vi "git resolve conflicts command.vi"(10 "Choosen file":string, 11 "ours vi path":path) -> (2 "git stage file and resolve conflict":string, 3 "git checkout selected file cmd":string)   [LabVIEW 2022 SP3]
panel:
  # "This is the path of the repository on which we are resolving conflicts. In this path needs to be \"ours\" repository."
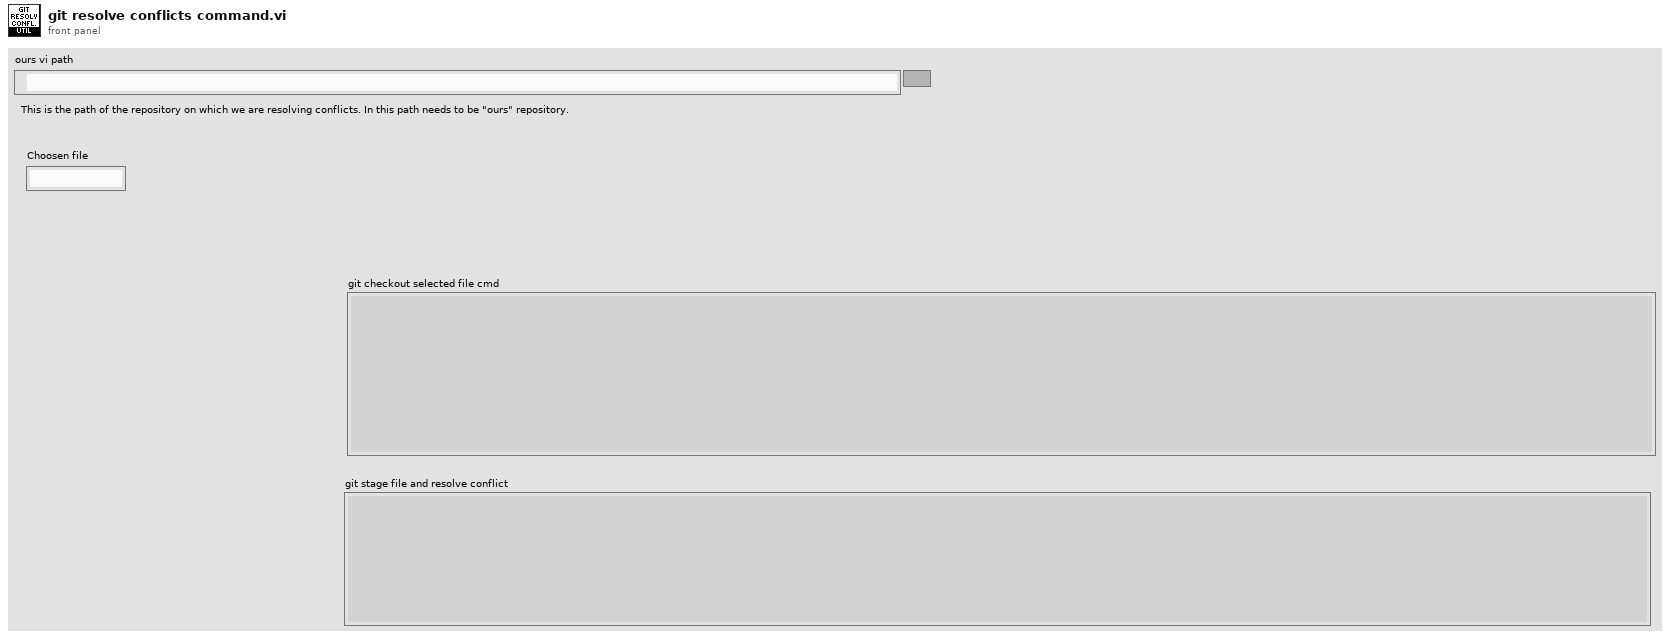
[diagram p1: front panel]
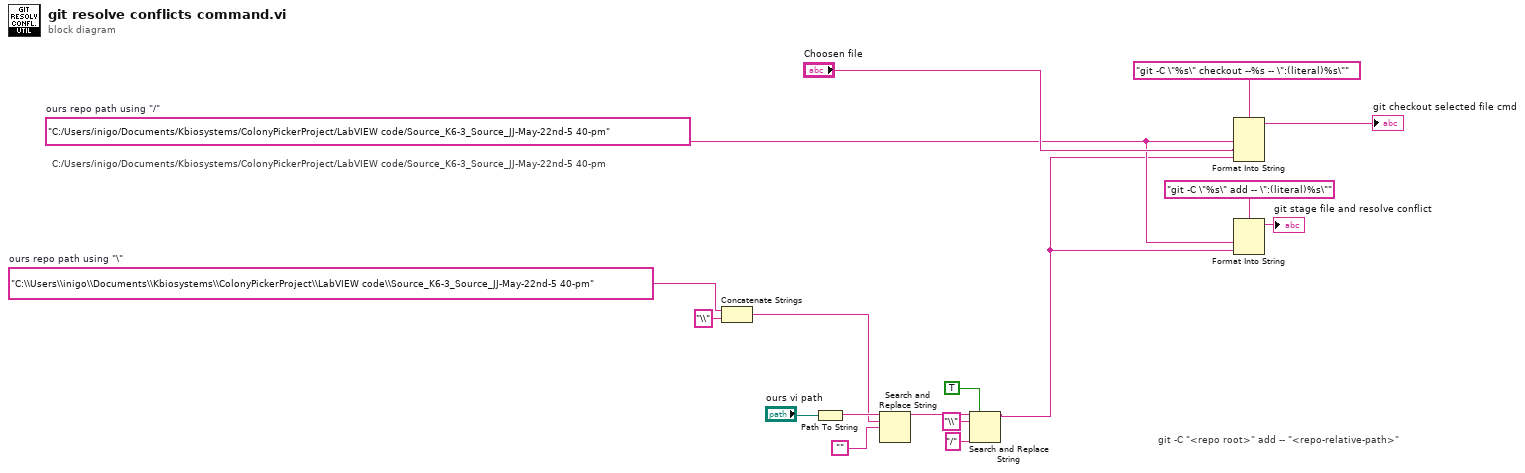
[diagram p0: block diagram]
diagram:
  w5 = "C:\\Users\\inigo\\Documents\\Kbiosystems\\ColonyPickerProject\\LabVIEW code\\Source_K6-3_Source_JJ-May-22nd-5 40-pm"  # ours repo path using "\"
  w3 = "C:/Users/inigo/Documents/Kbiosystems/ColonyPickerProject/LabVIEW code/Source_K6-3_Source_JJ-May-22nd-5 40-pm"  # ours repo path using "/"
  # "git -C \"<repo root>\" add -- \"<repo-relative-path>\""
  # "C:/Users/inigo/Documents/Kbiosystems/ColonyPickerProject/LabVIEW code/Source_K6-3_Source_JJ-May-22nd-5 40-pm"
  n1 = Concatenate Strings(w5, "\\" ("string")) -> (w9:string)
  n2 = Path To String(path="ours vi path") -> (string=w16:string)
  n3 = Search and Replace String(input string=w16, search string=w9, replace string="") -> (result string=w14:string)  [unwired: 5 in, 3 out]
  n4 = Search and Replace String(replace all?=TRUE ("replace all? (F)"), input string=w14, search string="\\", replace string="/" ("replace string (\"\")")) -> (result string=w2:string)  [unwired: 4 in, 3 out]
  n5 = Format Into String(format string="git -C \"%s\" checkout --%s -- \":(literal)%s\"", w3, "Choosen file", w2) -> (resulting string=→"git checkout selected file cmd":string)  [unwired: 2 in, 1 out]
  n6 = Format Into String(format string="git -C \"%s\" add -- \":(literal)%s\"", w3, w2) -> (resulting string=→"git stage file and resolve conflict":string)  [unwired: 2 in, 1 out]
